vi "uTTA_GV_Serial_Monitor.vi"() -> ()   [LabVIEW 2021]
panel:
  in  "Buffer Length":u32=1024
  out "Enabled":bool
  out "Serial Monitor":string
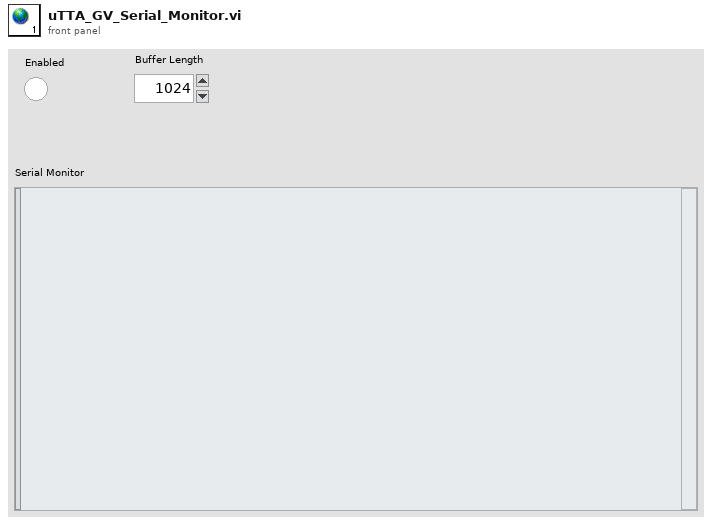
[diagram p1: front panel]
diagram:
